vi "Set SA Path.vi"(0 "SA Path in":refnum<class "SA Path.lvclass">, 11 "error in":errorcluster) -> (4 "SA Path out":refnum<class "SA Path.lvclass">, 15 "error out":errorcluster)   [LabVIEW 2023, in "RFFixtureCharact.RMM.lvlib" / "SA Path.lvclass"]
uses:
  SA Path.lvclass
  C:/srd-semi-rfcal-software - Main/AuxTools/STSRFFixtureCharactUtility/Source/Code Modules/Fixture/Public/Base Classes/Scalar/SA Abstract Path/SA Abstract Path.lvclass
  C:/srd-semi-rfcal-software - Main/AuxTools/STSRFFixtureCharactUtility/Source/Code Modules/Common/Base Classes/Path/Path.lvclass
  Public/Base Classes/Scalar/SA Abstract Path/SA Abstract Path.lvclass/SA Abstract Path.ctl
  Public/Base Classes/Scalar/SA Abstract Path/Properties/Read RFmx Session.vi
  Public/Base Classes/Scalar/SA Path/SA Path.lvclass
  SA Path.lvclass/SA Path.ctl
  <resource>/objmgr/RFmxSpecAn.rc
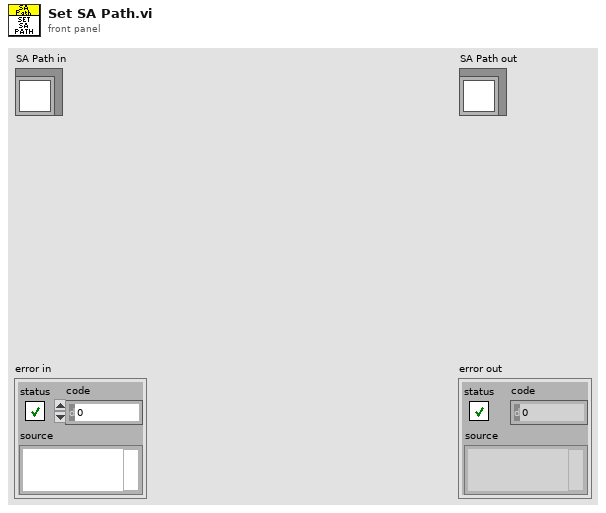
[diagram p1: front panel]
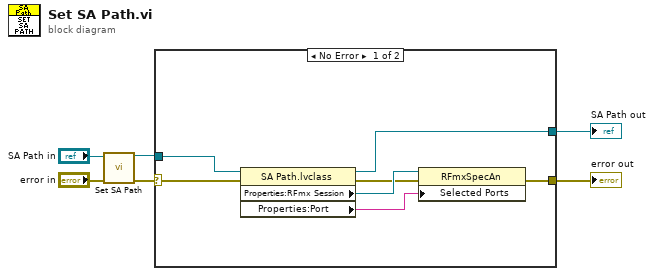
[diagram p0: block diagram]
diagram:
  n1 = call-parent "Set SA Path.vi"("SA Path in"="SA Path in", "error in (no error)"="error in") -> ("SA Path out"=w2:refnum<class "SA Path.lvclass">, "error out"=w4:errorcluster)  [unwired: 12 in]
  n2 = case shown="No Error" w4 {
    selector: w4 -> [w13 w15]
    tunnel: w2 -> [w12 w14]
    tunnel: [w11 w14] -> w6
    tunnel: [w8 w15] -> w5
    frame No Error {
      n3 = property class="SA Path.lvclass"(reference=w12, error in=w13) -> (reference out=w11:refnum<class "SA Path.lvclass">, error out=w9:errorcluster, "Properties:RFmx Session"=w10:refnum<k21>, "Properties:Port"=w7:string)
      n4 = property class="RFmxSpecAn"(reference=w10, error in=w9, "Selected Ports"=w7) -> (error out=w8:errorcluster)  [unwired: 1 out]
    }
    frame Error {
    }
  }
  "error out" <- w5
  "SA Path out" <- w6
